vi "XYZ Data.vi"() -> (0 "XYZ Stage Data":T1={"Configuration"={"Connection Settings"={"Tango VISA"="", "Baudrate"=57600, "Show Protocol?"=FALSE}, "Manual Control"={"North"=FALSE, "South"=FALSE, "West"=FALSE, "East"=FALSE, "Up"=FALSE, "Down"=FALSE, "Stop"=FALSE, "XY Step"=0.0, "Z step"=0.0}, "Coordinate Control"={"Motion Mode"=enum."Absolute", "Destination [mm]"=[]}}, "Refnums"={"Instrument Status"=refnum, "Position"=refnum, "Manual Control"=refnum, "Up"=refnum, "Down"=refnum, "North"=refnum, "South"=refnum, "East"=refnum, "West"=refnum, "Stop"=refnum, "Limits"=refnum}, "Initialization"={"Update Visa Session"=FALSE, "Set To Default"=FALSE, "Get Status"=FALSE, "Update Refnums"=FALSE}} {"Configuration"."Manual Control"."Z step" scale=0.1..10.0; "Configuration"."Manual Control"."XY Step" scale=0.1..1000.0})   [LabVIEW 2014]
uses:
  XYZ Data.ctl
  XYZ Config.ctl
  XYZ Connection Settings.ctl
  XYZ Stage Control.ctl
  XYZ Coordinate Control.ctl
  XYZ Refnums.ctl
  support/Instrument Status.ctl
  <instrlib>/Tango Drivers/Labview/SubVIs/Axis_Switch.ctl
  XYZ Initialization.ctl
panel:
  # "LICENSED MATERIALS – PROPERTY OF IBM\nCopyright IBM Corp. 2016,\nALL RIGHTS RESERVED"
  # "XY"
  # "Z"
  # "XY"
  # "Z"
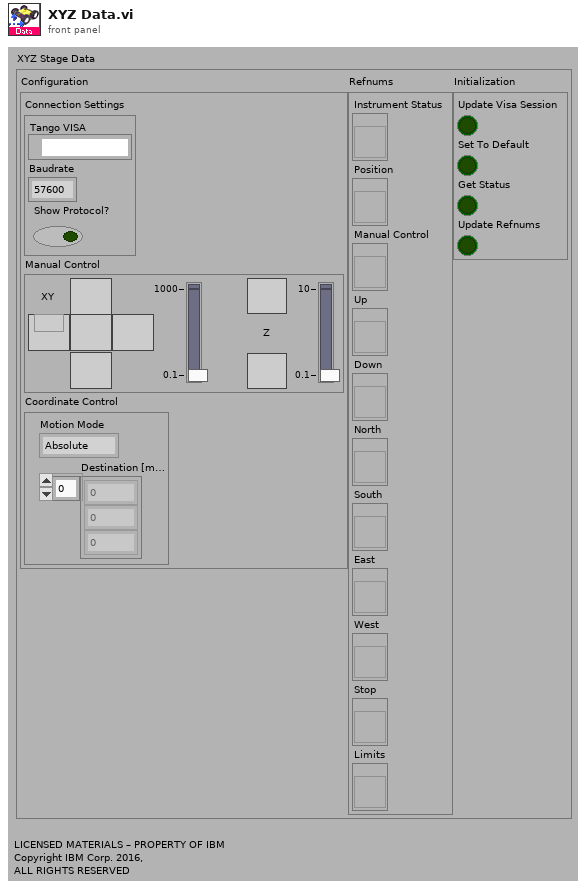
[diagram p1: front panel]
types:
  T1 = typedef "XYZ Data.ctl" = cluster{"Configuration":T2, "Refnums":T6, "Initialization":T7}
  T2 = typedef "XYZ Config.ctl" = cluster{"Connection Settings":T3, "Manual Control":T4, "Coordinate Control":T5}
  T3 = typedef "XYZ Connection Settings.ctl" = cluster{"Tango VISA":refnum<visa-resource-name>, "Baudrate":i32, "Show Protocol?":bool}
  T4 = typedef "XYZ Stage Control.ctl" = cluster{"North":bool, "South":bool, "West":bool, "East":bool, "Up":bool, "Down":bool, "Stop":bool, "XY Step":dbl, "Z step":dbl}
  T5 = typedef "XYZ Coordinate Control.ctl" = cluster{"Motion Mode":enum16{"Absolute", "Relative"}, "Destination [mm]":dbl[]}
  T6 = typedef "XYZ Refnums.ctl" = cluster{"Instrument Status":refnum<vi>, "Position":refnum<vi>, "Manual Control":refnum<vi>, "Up":refnum<vi>, "Down":refnum<vi>, "North":refnum<vi>, "South":refnum<vi>, "East":refnum<vi>, "West":refnum<vi>, "Stop":refnum<vi>, "Limits":refnum<vi>}
  T7 = typedef "XYZ Initialization.ctl" = cluster{"Update Visa Session":bool, "Set To Default":bool, "Get Status":bool, "Update Refnums":bool}
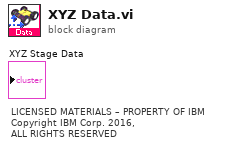
[diagram p0: block diagram]
diagram:
  # "LICENSED MATERIALS – PROPERTY OF IBM\nCopyright IBM Corp. 2016,\nALL RIGHTS RESERVED"
